vi "Emergency message into error.vi"(1 "emergency message":T1 {"manufacturer specific error field" format="%.0x"; "error register" format="%.0x"; "error code" format="%.0x"}) -> (0 "error":errorcluster)   [LabVIEW 2016]
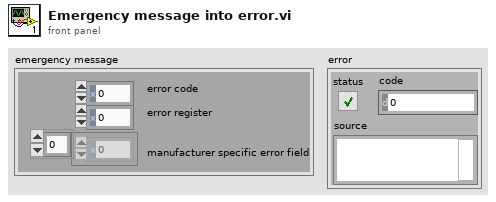
[diagram p1: front panel]
types:
  T1 = cluster{"error code":u16, "error register":u8, "manufacturer specific error field":u8[]}
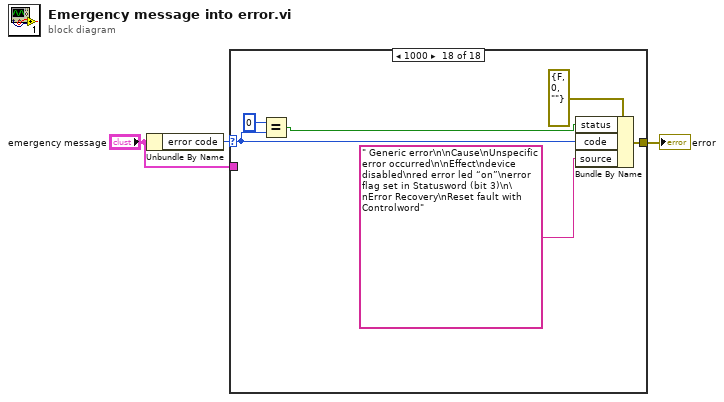
[diagram p0: block diagram]
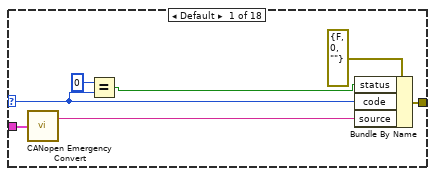
[diagram p2: hidden frame]
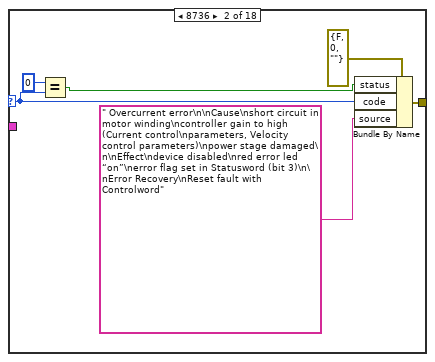
[diagram p3: hidden frame]
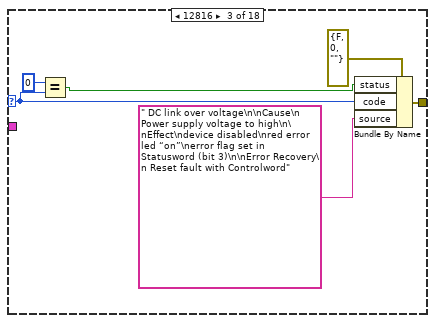
[diagram p4: hidden frame]
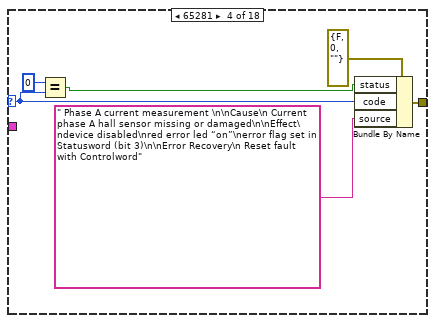
[diagram p5: hidden frame]
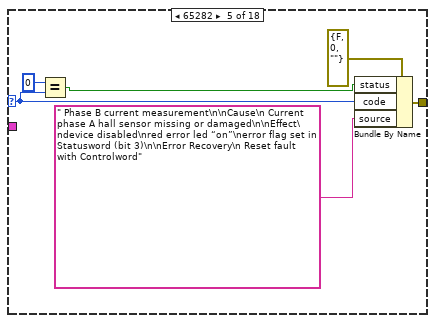
[diagram p6: hidden frame]
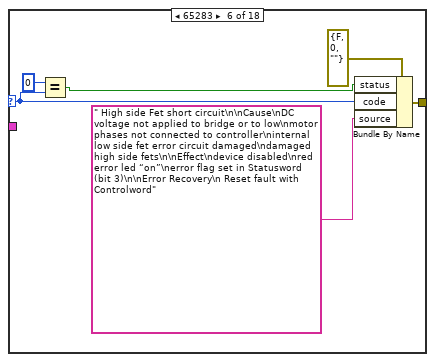
[diagram p7: hidden frame]
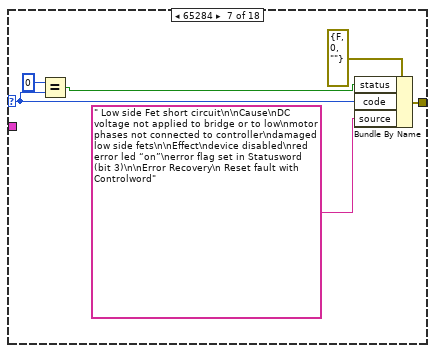
[diagram p8: hidden frame]
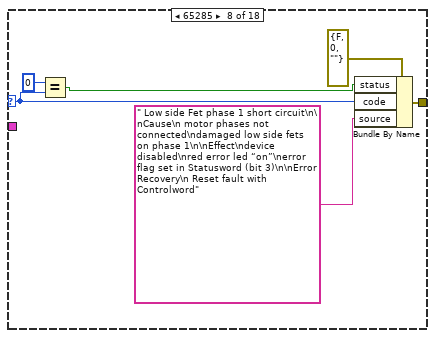
[diagram p9: hidden frame]
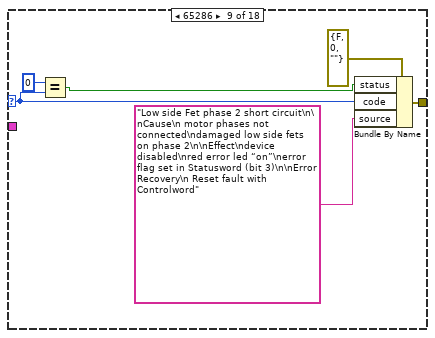
[diagram p10: hidden frame]
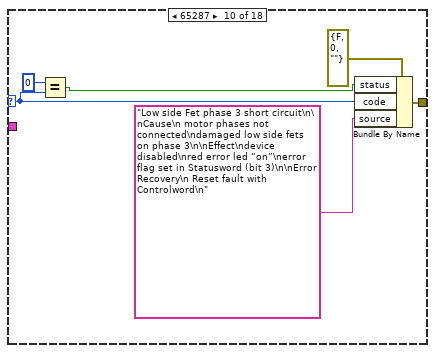
[diagram p11: hidden frame]
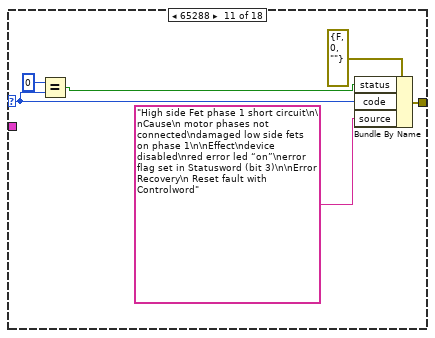
[diagram p12: hidden frame]
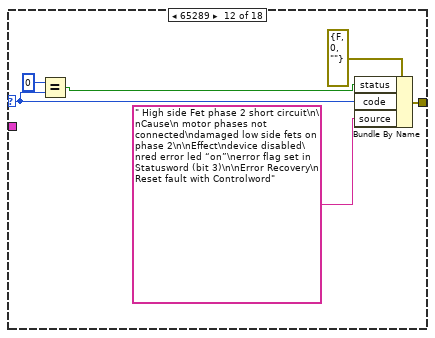
[diagram p13: hidden frame]
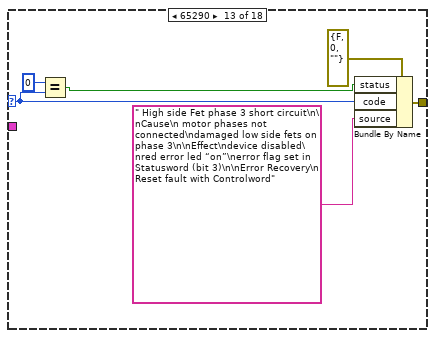
[diagram p14: hidden frame]
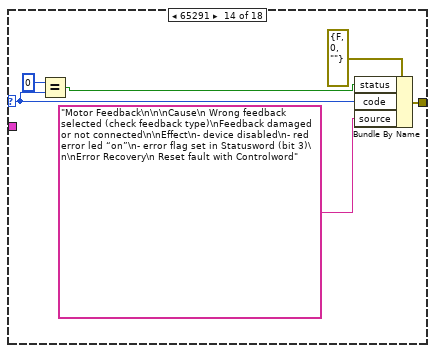
[diagram p15: hidden frame]
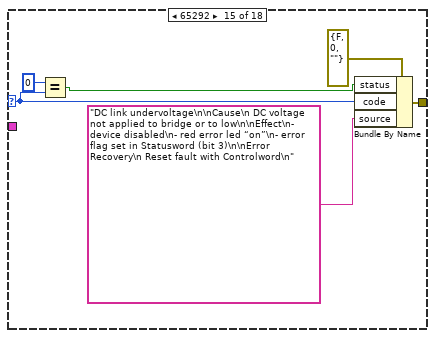
[diagram p16: hidden frame]
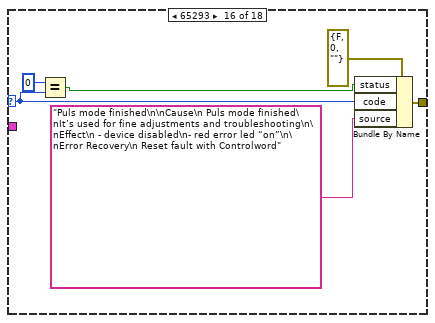
[diagram p17: hidden frame]
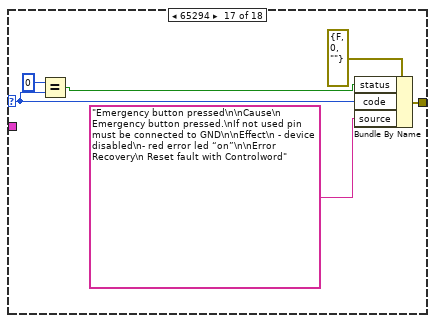
[diagram p18: hidden frame]
diagram:
  n1 = Unbundle By Name("emergency message") -> ("error code"=w2:u16)
  n2 = case shown="1000" w2 {
    selector: w2 -> [w8 w12 w18 w24 w30 w36 w42 w48 w54 w60 w66 w71 w78 w84 w90 w96 w105 w107]
    tunnel: [w9 w11 w17 w23 w29 w35 w41 w47 w53 w59 w65 w72 w77 w83 w89 w95 w101 w108] -> w3
    tunnel: "emergency message" -> [w4 _ _ _ _ _ _ _ _ _ _ _ _ _ _ _ _ _]
    frame Default {
      n3 = call <vilib>:"CANopen Emergency Convert.vi"("emergency message"=w4) -> ("error description"=w5:string)  [unwired: 1 out]
      n4 = Equal?(x=u16 0, y=w8) -> (x = y?=w6:bool)
      n5 = Bundle By Name(cluster=errorcluster {"status"=FALSE, "code"=0, "source"=""} ("error constant"), "status"=w6, "code"=w8, "source"=w5) -> (w9:errorcluster)
    }
    frame 8736 {
      n6 = Equal?(x=u16 0, y=w12) -> (x = y?=w14:bool)
      n7 = Bundle By Name(cluster=errorcluster {"status"=FALSE, "code"=0, "source"=""} ("error constant"), "status"=w14, "code"=w12, "source"=" Overcurrent error\n\nCause\nshort circuit in motor winding\ncontroller gain to high (Current control\nparameters, Velocity control parameters)\npower stage damaged\n\nEffect\ndevice disabled\nred error led “on”\nerror flag set in Statusword (bit 3)\n\nError Recovery\nReset fault with Controlword") -> (w11:errorcluster)
    }
    frame 12816 {
      n8 = Equal?(x=u16 0, y=w18) -> (x = y?=w20:bool)
      n9 = Bundle By Name(cluster=errorcluster {"status"=FALSE, "code"=0, "source"=""} ("error constant"), "status"=w20, "code"=w18, "source"=" DC link over voltage\n\nCause\n Power supply voltage to high\n\nEffect\ndevice disabled\nred error led “on”\nerror flag set in Statusword (bit 3)\n\nError Recovery\n Reset fault with Controlword") -> (w17:errorcluster)
    }
    frame 65281 {
      n10 = Equal?(x=u16 0, y=w24) -> (x = y?=w26:bool)
      n11 = Bundle By Name(cluster=errorcluster {"status"=FALSE, "code"=0, "source"=""} ("error constant"), "status"=w26, "code"=w24, "source"=" Phase A current measurement \n\nCause\n Current phase A hall sensor missing or damaged\n\nEffect\ndevice disabled\nred error led “on”\nerror flag set in Statusword (bit 3)\n\nError Recovery\n Reset fault with Controlword") -> (w23:errorcluster)
    }
    frame 65282 {
      n12 = Equal?(x=u16 0, y=w30) -> (x = y?=w32:bool)
      n13 = Bundle By Name(cluster=errorcluster {"status"=FALSE, "code"=0, "source"=""} ("error constant"), "status"=w32, "code"=w30, "source"=" Phase B current measurement\n\nCause\n Current phase A hall sensor missing or damaged\n\nEffect\ndevice disabled\nred error led “on”\nerror flag set in Statusword (bit 3)\n\nError Recovery\n Reset fault with Controlword") -> (w29:errorcluster)
    }
    frame 65283 {
      n14 = Equal?(x=u16 0, y=w36) -> (x = y?=w38:bool)
      n15 = Bundle By Name(cluster=errorcluster {"status"=FALSE, "code"=0, "source"=""} ("error constant"), "status"=w38, "code"=w36, "source"=" High side Fet short circuit\n\nCause\nDC voltage not applied to bridge or to low\nmotor phases not connected to controller\ninternal low side fet error circuit damaged\ndamaged high side fets\n\nEffect\ndevice disabled\nred error led “on”\nerror flag set in Statusword (bit 3)\n\nError Recovery\n Reset fault with Controlword") -> (w35:errorcluster)
    }
    frame 65284 {
      n16 = Equal?(x=u16 0, y=w42) -> (x = y?=w44:bool)
      n17 = Bundle By Name(cluster=errorcluster {"status"=FALSE, "code"=0, "source"=""} ("error constant"), "status"=w44, "code"=w42, "source"=" Low side Fet short circuit\n\nCause\nDC voltage not applied to bridge or to low\nmotor phases not connected to controller\ndamaged low side fets\n\nEffect\ndevice disabled\nred error led “on”\nerror flag set in Statusword (bit 3)\n\nError Recovery\n Reset fault with Controlword") -> (w41:errorcluster)
    }
    frame 65285 {
      n18 = Equal?(x=u16 0, y=w48) -> (x = y?=w51:bool)
      n19 = Bundle By Name(cluster=errorcluster {"status"=FALSE, "code"=0, "source"=""} ("error constant"), "status"=w51, "code"=w48, "source"=" Low side Fet phase 1 short circuit\n\nCause\n motor phases not connected\ndamaged low side fets on phase 1\n\nEffect\ndevice disabled\nred error led “on”\nerror flag set in Statusword (bit 3)\n\nError Recovery\n Reset fault with Controlword") -> (w47:errorcluster)
    }
    frame 65286 {
      n20 = Equal?(x=u16 0, y=w54) -> (x = y?=w57:bool)
      n21 = Bundle By Name(cluster=errorcluster {"status"=FALSE, "code"=0, "source"=""} ("error constant"), "status"=w57, "code"=w54, "source"="Low side Fet phase 2 short circuit\n\nCause\n motor phases not connected\ndamaged low side fets on phase 2\n\nEffect\ndevice disabled\nred error led “on”\nerror flag set in Statusword (bit 3)\n\nError Recovery\n Reset fault with Controlword") -> (w53:errorcluster)
    }
    frame 65287 {
      n22 = Equal?(x=u16 0, y=w60) -> (x = y?=w62:bool)
      n23 = Bundle By Name(cluster=errorcluster {"status"=FALSE, "code"=0, "source"=""} ("error constant"), "status"=w62, "code"=w60, "source"="Low side Fet phase 3 short circuit\n\nCause\n motor phases not connected\ndamaged low side fets on phase 3\n\nEffect\ndevice disabled\nred error led “on”\nerror flag set in Statusword (bit 3)\n\nError Recovery\n Reset fault with Controlword\n") -> (w59:errorcluster)
    }
    frame 65288 {
      n24 = Equal?(x=u16 0, y=w66) -> (x = y?=w69:bool)
      n25 = Bundle By Name(cluster=errorcluster {"status"=FALSE, "code"=0, "source"=""} ("error constant"), "status"=w69, "code"=w66, "source"="High side Fet phase 1 short circuit\n\nCause\n motor phases not connected\ndamaged low side fets on phase 1\n\nEffect\ndevice disabled\nred error led “on”\nerror flag set in Statusword (bit 3)\n\nError Recovery\n Reset fault with Controlword") -> (w65:errorcluster)
    }
    frame 65289 {
      n26 = Equal?(x=u16 0, y=w71) -> (x = y?=w74:bool)
      n27 = Bundle By Name(cluster=errorcluster {"status"=FALSE, "code"=0, "source"=""} ("error constant"), "status"=w74, "code"=w71, "source"=" High side Fet phase 2 short circuit\n\nCause\n motor phases not connected\ndamaged low side fets on phase 2\n\nEffect\ndevice disabled\nred error led “on”\nerror flag set in Statusword (bit 3)\n\nError Recovery\n Reset fault with Controlword") -> (w72:errorcluster)
    }
    frame 65290 {
      n28 = Equal?(x=u16 0, y=w78) -> (x = y?=w81:bool)
      n29 = Bundle By Name(cluster=errorcluster {"status"=FALSE, "code"=0, "source"=""} ("error constant"), "status"=w81, "code"=w78, "source"=" High side Fet phase 3 short circuit\n\nCause\n motor phases not connected\ndamaged low side fets on phase 3\n\nEffect\ndevice disabled\nred error led “on”\nerror flag set in Statusword (bit 3)\n\nError Recovery\n Reset fault with Controlword") -> (w77:errorcluster)
    }
    frame 65291 {
      n30 = Equal?(x=u16 0, y=w84) -> (x = y?=w86:bool)
      n31 = Bundle By Name(cluster=errorcluster {"status"=FALSE, "code"=0, "source"=""} ("error constant"), "status"=w86, "code"=w84, "source"="Motor Feedback\n\n\nCause\n Wrong feedback selected (check feedback type)\nFeedback damaged or not connected\n\nEffect\n- device disabled\n- red error led “on”\n- error flag set in Statusword (bit 3)\n\nError Recovery\n Reset fault with Controlword") -> (w83:errorcluster)
    }
    frame 65292 {
      n32 = Equal?(x=u16 0, y=w90) -> (x = y?=w92:bool)
      n33 = Bundle By Name(cluster=errorcluster {"status"=FALSE, "code"=0, "source"=""} ("error constant"), "status"=w92, "code"=w90, "source"="DC link undervoltage\n\nCause\n DC voltage not applied to bridge or to low\n\nEffect\n- device disabled\n- red error led “on”\n- error flag set in Statusword (bit 3)\n\nError Recovery\n Reset fault with Controlword\n") -> (w89:errorcluster)
    }
    frame 65293 {
      n34 = Equal?(x=u16 0, y=w96) -> (x = y?=w98:bool)
      n35 = Bundle By Name(cluster=errorcluster {"status"=FALSE, "code"=0, "source"=""} ("error constant"), "status"=w98, "code"=w96, "source"="Puls mode finished\n\nCause\n Puls mode finished\nIt’s used for fine adjustments and troubleshooting\n\nEffect\n - device disabled\n- red error led “on”\n\nError Recovery\n Reset fault with Controlword") -> (w95:errorcluster)
    }
    frame 65294 {
      n36 = Equal?(x=u16 0, y=w105) -> (x = y?=w103:bool)
      n37 = Bundle By Name(cluster=errorcluster {"status"=FALSE, "code"=0, "source"=""} ("error constant"), "status"=w103, "code"=w105, "source"="Emergency button pressed\n\nCause\n Emergency button pressed.\nIf not used pin must be connected to GND\n\nEffect\n - device disabled\n- red error led “on”\n\nError Recovery\n Reset fault with Controlword") -> (w101:errorcluster)
    }
    frame 4096 {
      n38 = Equal?(x=u16 0, y=w107) -> (x = y?=w110:bool)
      n39 = Bundle By Name(cluster=errorcluster {"status"=FALSE, "code"=0, "source"=""} ("error constant"), "status"=w110, "code"=w107, "source"=" Generic error\n\nCause\nUnspecific error occurred\n\nEffect\ndevice disabled\nred error led “on”\nerror flag set in Statusword (bit 3)\n\nError Recovery\nReset fault with Controlword") -> (w108:errorcluster)
    }
  }
  "error" <- w3
